vi "pionowy.vi"(6 "error in":errorcluster, 7 "Wybór komory":T1, 8 "Akcja":T8=enum."Reset ramienia", 9 "LINX Resource in":T2) -> (0 "error out":errorcluster, 1 "KONIEC":bool, 2 "Aktualny stan":T9, 3 "LINX Resource out":T2)   [LabVIEW 2014]
uses:
  pionowyVIs/RuchPionowy.ctl
  AkcjaRuchu.ctl
  <vilib>/MakerHub/LINX/Private/Type Defs/LINX Ref.ctl
  <vilib>/MakerHub/LINX/Private/Type Defs/Platform.ctl
  <vilib>/MakerHub/LINX/Private/Type Defs/Interface.ctl
  <vilib>/MakerHub/LINX/Private/Device/Type Defs/LINX Device Config.ctl
  <vilib>/MakerHub/LINX/Private/Device/Type Defs/TCP Config.ctl
  <vilib>/MakerHub/LINX/Private/Device/Type Defs/Channels.ctl
  parametryKomorVIs/WyborKomory.ctl
  Faza_ruchu.ctl
  pionowyVIs/ParametryRuchyPionowego.ctl
  pionowyVIs/usrednianieVIs/AkcjaUsredniania.ctl
  AkcjaGFV.ctl
  poziomyVIs/timerRuchuPoziomegoVIs/Czynnosc.ctl
  <vilib>/MakerHub/LINX/LMH-LINX.lvlib
  <vilib>/MakerHub/LINX/Private/Device/Device.lvlib
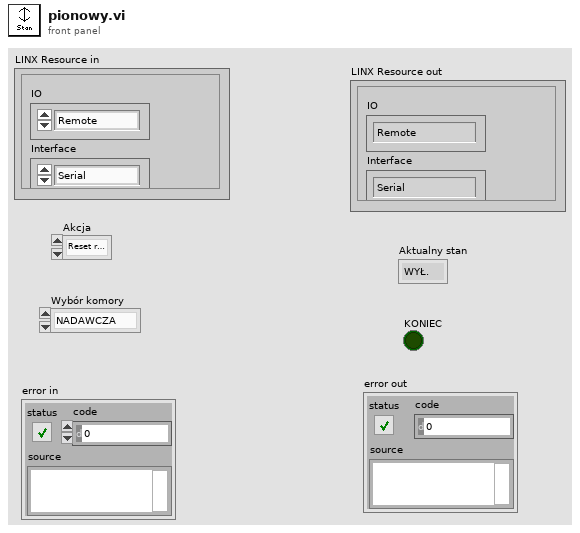
[diagram p1: front panel]
types:
  T1 = typedef "WyborKomory.ctl" = enum16{"NADAWCZA", "ODBIORCZA"}
  T2 = typedef "LMH-LINX.lvlib/LINX Ref.ctl" = cluster{"IO":T3, "Interface":T4, "LINX Device Config":T5}
  T3 = typedef "LMH-LINX.lvlib/Platform.ctl" = enum16{"Remote", "Local"}
  T4 = typedef "LMH-LINX.lvlib/Interface.ctl" = enum16{"Serial", "TCP"}
  T5 = typedef "LMH-LINX.lvlib/Device.lvlib/LINX Device Config.ctl" = cluster{"Interface":T4, "COM Port":refnum<visa-resource-name>, "TCP Configuration":T6, "Device Family":u8, "Device ID":u8, "Device Name":string, "TCP Ref":refnum<k5>, "Channels":T7}
  T6 = typedef "LMH-LINX.lvlib/Device.lvlib/TCP Config.ctl" = cluster{"IP Address":string, "Port":u16}
  T7 = typedef "LMH-LINX.lvlib/Channels.ctl" = cluster{"DI":u8[], "DO":u8[], "AI":u8[], "AO":u8[], "PWM":u8[], "QE":u8[], "UART":u8[], "I2C 2":u8[], "SPI":u8[], "CAN":u8[], "Servo":u8[], "AI Ref (V)":dbl, "AI Resolution (Bits)":u8, "AO Ref (V)":dbl, "AO Resolution (Bits)":u8}
  T8 = typedef "AkcjaRuchu.ctl" = enum16{"Init", "Reset ramienia", "Przygotuj listę", "Sprawdź", "Koniec"}
  T9 = typedef "RuchPionowy.ctl" = enum16{"WYŁ.", "GÓRA", "Dӣ", "PRACA RĘCZNA"}
  T10 = typedef "Czynnosc.ctl" = enum16{"reset all", "działaj"}
  T11 = typedef "AkcjaGFV.ctl" = enum16{"Czytaj", "Zapisz", "Reset"}
  T12 = typedef "AkcjaUsredniania.ctl" = enum16{"Init", "DodajWartość", "OdczytajPrzyspieszenie", "WypełnijKolejkę", "Czyść"}
  T13 = typedef "ParametryRuchyPionowego.ctl" = cluster{"Faza ruchu":T14, "Lista punktów w pionie":i32[]}
  T14 = typedef "Faza_ruchu.ctl" = enum16{"Ruch", "Poczekaj", "Pomiar"}
  T15 = typedef "Gotowosc.ctl" = cluster{"Poziomy":bool, "Pionowy":bool}
  T16 = typedef "WejsciaParametry.ctl" = cluster{"LEWO":bool, "PRAWO":bool, "GORA":bool, "DOL":bool, "Praca reczna":bool, "Stop":bool, "Start":bool, "Komora":bool, "Wyjscie":bool, "Rodzaj pomiarow":T17, "Czas pomiaru [s]":dbl, "Czas inicjalizacji ramion [s]":dbl, "Liczba punktów":i32, "Liczba płaszczyzn":i32}
  T17 = typedef "RodzajPomiarow.ctl" = enum16{"Izolacyjność Akustyczna ISO 10140", "Losowanie punktów", "Sekwencja testowa"}
  T18 = typedef "WyjsciaParametry.ctl" = cluster{"Nad. lewo":bool, "Nad.  prawo":bool, "Nad.  gora":bool, "Nad. doł":bool, "Dzialanie":bool, "Pomiar":bool, "Odb. lewo":bool, "Odb.  prawo":bool, "Odb.  gora":bool, "Odb. dol":bool, "Pozostalo punktow":i32, "Nad. elewacja":i32, "Nad. azymut":i32, "Odb. elewacja":i32, "Odb. azymut":i32, "TCP Error":bool, "TCP Error Code":i32, "LINX Error":bool, "LINX Error Code":i32, "Nastepny elewacja":i32, "Nastepny azymut":i32, "Coords Error":bool, "Inicjalizacja pozycji":bool}
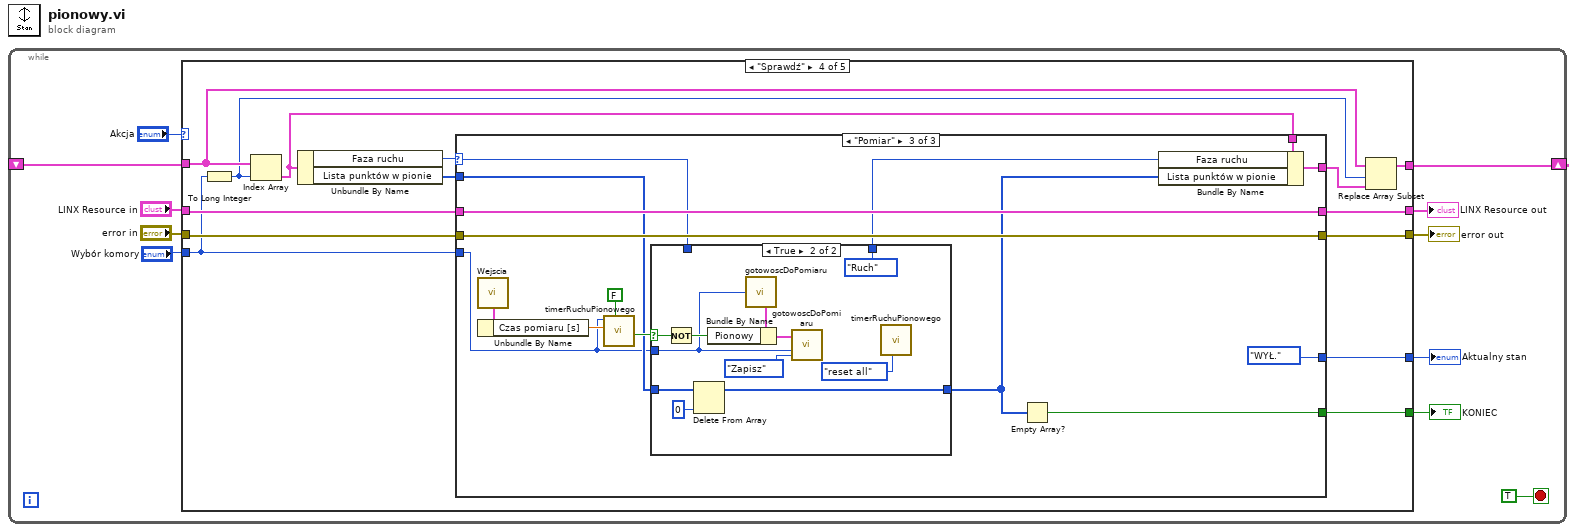
[diagram p0: block diagram]
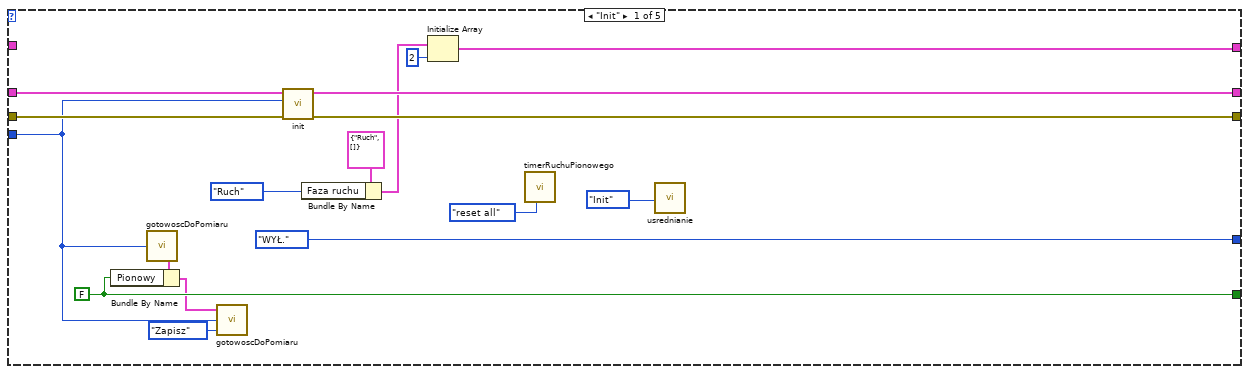
[diagram p2: hidden frame]
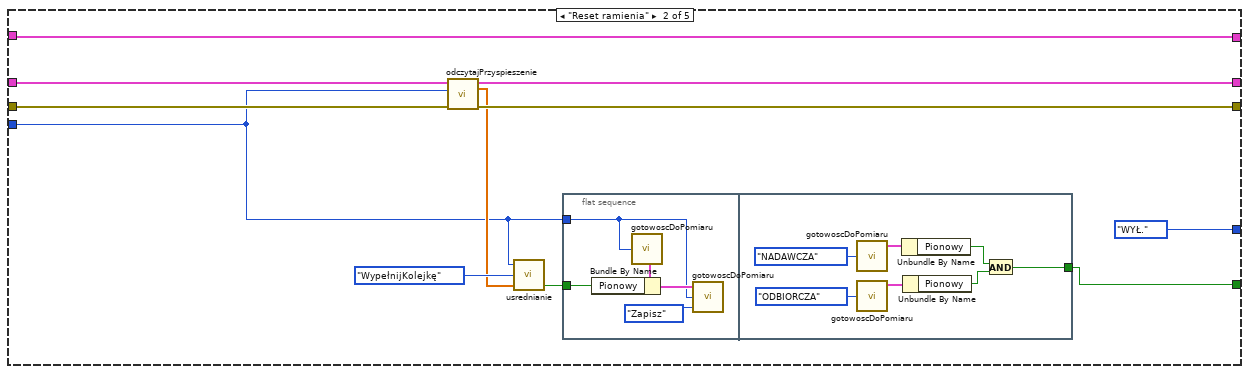
[diagram p3: hidden frame]
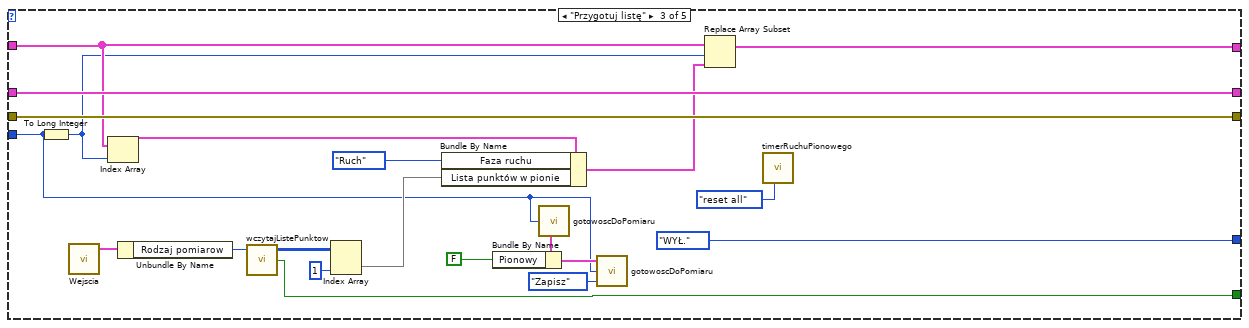
[diagram p4: hidden frame]
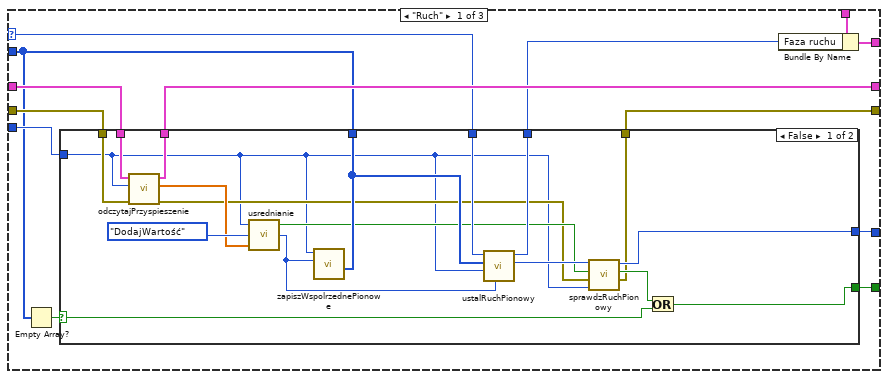
[diagram p5: hidden frame]
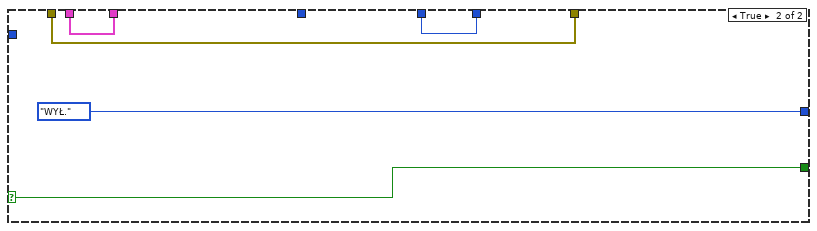
[diagram p6: hidden frame]
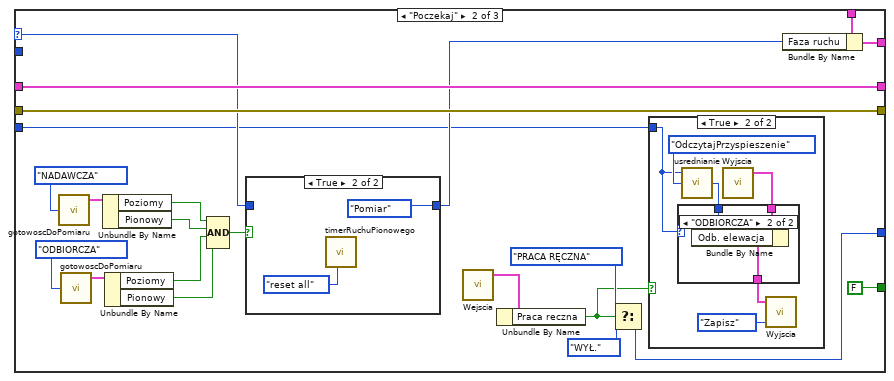
[diagram p7: hidden frame]
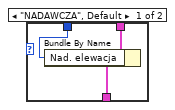
[diagram p9: hidden frame]
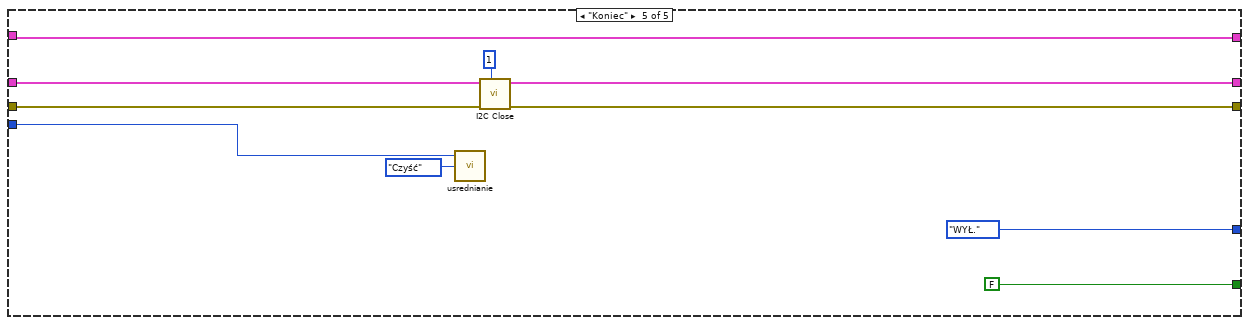
[diagram p12: hidden frame]
diagram:
  n1 = while {
    shift-right: [w10] -> _
    shift-left: _ -> [w7]
    stop <- TRUE stop-if-true
    n2 = case shown="\"Sprawdź\"" "Akcja" {
      tunnel: "error in" -> [w26 w36 w71 w85 w196]
      tunnel: [w24 w34 w71 w83 w193] -> w3
      tunnel: [w25 w35 w72 w84 w194] -> w4
      tunnel: "LINX Resource in" -> [w27 w37 w72 w86 w197]
      tunnel: [w16 w30 w53 w81 FALSE ("empty?")] -> w1
      tunnel: [RuchPionowy."WYŁ." ("Aktualny stan") RuchPionowy."WYŁ." ("Aktualny stan") RuchPionowy."WYŁ." ("Aktualny stan") w82 RuchPionowy."WYŁ." ("Aktualny stan")] -> w2
      tunnel: "Wybór komory" -> [w13 w29 w55 w80 w189]
      tunnel: [w18 w32 w68 w76 w188] -> w10
      tunnel: w7 -> [_ w32 w65 w77 w188]
      frame "Init" {
        w16 = FALSE ("Poziomy")
        n3 = call "gotowoscDoPomiaru.vi"("Wybór komory"=w13) -> ("Gotowość wyjście"=w17:T15)  [unwired: 4 in]
        n4 = Bundle By Name(cluster=w17, "Pionowy"=w16) -> (w15:T15)
        n5 = call "gotowoscDoPomiaru.vi"("Akcja"=AkcjaGFV."Zapisz", "Wybór komory"=w13, "Gotowość"=w15) -> ()  [unwired: 2 in, 1 out]
        n6 = call "init.vi"("Error In"=w26, "Wybór komory"=w13, "LINX Ref"=w27) -> ("Error Out"=w24:errorcluster, "LINX Resource"=w25:T2)  [unwired: 7 in]
        n7 = Bundle By Name(cluster=T13 {"Faza ruchu"=enum."Ruch", "Lista punktów w pionie"=[]} ("Parametry ruchy pionowego"), "Faza ruchu"=Faza_ruchu."Ruch") -> (w20:T13)
        n8 = Initialize Array(w20, 2 ("dimension size")) -> (w18:T13[])
        n9 = call "timerRuchuPionowego.vi"("Czynność"=Czynnosc."reset all") -> ()  [unwired: 10 in, 1 out]
        n10 = call "usrednianie.vi"("AkcjaUsredniania"=AkcjaUsredniania."Init") -> ()  [unwired: 2 in, 3 out]
      }
      frame "Reset ramienia" {
        n11 = call "odczytajPrzyspieszenie.vi"("Error In"=w36, "Wybór komory"=w29, "LINX Resource"=w37) -> ("Error Out"=w34:errorcluster, "Kąty nachylenia (st.)"=w33:dbl[], "LINX Resource 2"=w35:T2)  [unwired: 6 in]
        n12 = call "usrednianie.vi"("Wartości"=w33, "AkcjaUsredniania"=AkcjaUsredniania."WypełnijKolejkę", "Wybór Komory"=w29) -> ("Czy kolejka pełna?"=w31:bool)  [unwired: 2 out]
        n13 = flat-sequence {
          tunnel: w31 -> [w41]
          tunnel: w29 -> [w40]
          tunnel: [w45] -> w30
          frame #0 {
            n14 = call "gotowoscDoPomiaru.vi"("Wybór komory"=w40) -> ("Gotowość wyjście"=w44:T15)  [unwired: 4 in]
            n15 = Bundle By Name(cluster=w44, "Pionowy"=w41) -> (w43:T15)
            n16 = call "gotowoscDoPomiaru.vi"("Akcja"=AkcjaGFV."Zapisz", "Wybór komory"=w40, "Gotowość"=w43) -> ()  [unwired: 2 in, 1 out]
          }
          frame #1 {
            n17 = call "gotowoscDoPomiaru.vi"("Wybór komory"=WyborKomory."NADAWCZA") -> ("Gotowość wyjście"=w48:T15)  [unwired: 4 in]
            n18 = call "gotowoscDoPomiaru.vi"("Wybór komory"=WyborKomory."ODBIORCZA") -> ("Gotowość wyjście"=w49:T15)  [unwired: 4 in]
            n19 = Unbundle By Name(w48) -> ("Pionowy"=w51:bool)
            n20 = Unbundle By Name(w49) -> ("Pionowy"=w50:bool)
            n21 = And(x=w51, y=w50) -> (x .and. y?=w45:bool)
          }
        }
      }
      frame "Przygotuj listę" {
        n22 = To Long Integer(number=w55) -> (32bit integer=w56:i32)
        n23 = call "Wejscia.vi"() -> ("Wyjście"=w61:T16)  [unwired: 5 in]
        n24 = Index Array(array=w65, index=w56) -> (element=w66:T13)
        n25 = Unbundle By Name(w61) -> ("Rodzaj pomiarow"=w60:T17)
        n26 = call "wczytajListePunktow.vi"("Rodzaj pomiarow"=w60) -> ("Blad"=w53:bool, "Wspolrzedne katowe"=w64:i32[][])  [unwired: 3 in]
        n27 = Index Array(array=w64, index (col)=1 ("disabled index (col)")) -> (element=w62:i32[])  [unwired: 1 in]
        n28 = Bundle By Name(cluster=w66, "Faza ruchu"=Faza_ruchu."Ruch", "Lista punktów w pionie"=w62) -> (w67:T13)
        n29 = call "gotowoscDoPomiaru.vi"("Wybór komory"=w55) -> ("Gotowość wyjście"=w59:T15)  [unwired: 4 in]
        n30 = Bundle By Name(cluster=w59, "Pionowy"=FALSE ("Poziomy")) -> (w58:T15)
        n31 = call "gotowoscDoPomiaru.vi"("Akcja"=AkcjaGFV."Zapisz", "Wybór komory"=w55, "Gotowość"=w58) -> ()  [unwired: 2 in, 1 out]
        n32 = Replace Array Subset(array=w65, new element=w67, index=w56) -> (w68:T13[])
        n33 = call "timerRuchuPionowego.vi"("Czynność"=Czynnosc."reset all") -> ()  [unwired: 10 in, 1 out]
      }
      frame "Sprawdź" {
        n34 = To Long Integer(number=w80) -> (32bit integer=w74:i32)
        n35 = Index Array(array=w77, index=w74) -> (element=w73:T13)
        n36 = Unbundle By Name(w73) -> ("Faza ruchu"=w79:T14, "Lista punktów w pionie"=w78:i32[])
        n37 = case shown="\"Pomiar\"" w79 {
          selector: w79 -> [w94 w142 w169]
          tunnel: w86 -> [w98 w144 w174]
          tunnel: w85 -> [w99 w143 w173]
          tunnel: [w96 w143 w173] -> w83
          tunnel: [w97 w144 w174] -> w84
          tunnel: [w95 w139 RuchPionowy."WYŁ." ("Stan pionowy")] -> w82
          tunnel: [w92 FALSE ("empty?") w168] -> w81
          tunnel: w80 -> [w91 w123 w160]
          tunnel: w78 -> [w88 _ w167]
          tunnel: [w89 w135 w164] -> w75
          tunnel: w73 -> [w87 w134 w163]
          frame "Ruch" {
            n38 = Empty Array?(array=w88) -> (empty?=w93:bool)
            n39 = case shown="False" w93 {
              selector: w93 -> [w105 w118]
              tunnel: w99 -> [w114 w121]
              tunnel: w98 -> [w112 w122]
              tunnel: [w113 w122] -> w97
              tunnel: [w102 w121] -> w96
              tunnel: [w107 RuchPionowy."WYŁ." ("Stan pionowy")] -> w95
              tunnel: w94 -> [w116 w120]
              tunnel: [w115 w120] -> w90
              tunnel: [w104 w118] -> w92
              tunnel: w91 -> [w100 _]
              tunnel: w88 -> [w110 _]
              frame False {
                n40 = call "odczytajPrzyspieszenie.vi"("Error In"=w114, "Wybór komory"=w100, "LINX Resource"=w112) -> ("Error Out"=w103:errorcluster, "Kąty nachylenia (st.)"=w111:dbl[], "LINX Resource 2"=w113:T2)  [unwired: 6 in]
                n41 = call "usrednianie.vi"("Wartości"=w111, "AkcjaUsredniania"=AkcjaUsredniania."DodajWartość", "Wybór Komory"=w100) -> ("Kąt uśredniony"=w101:i32, "Czy nastapil krok?"=w108:bool)  [unwired: 1 out]
                n42 = call "zapiszWspolrzednePionowe.vi"("Lista punktów w pionie"=w110, "Kąt uśredniony"=w101, "Wybór komory"=w100) -> ()  [unwired: 9 in]
                n43 = call "ustalRuchPionowy.vi"("Kąt uśredniony"=w101, "Wybór komory"=w100, "Lista punktów w pionie"=w110, "Faza ruchu wstepna"=w116) -> ("Stan pionowy"=w109:T9, "Faza ruchu poziomego"=w115:T14)  [unwired: 6 in]
                n44 = call "sprawdzRuchPionowy.vi"("Wybór komory"=w100, "LINX Error IN"=w103, "Czy nastapil krok?"=w108, "Stan pionowy"=w109) -> ("LINX Error OUT"=w102:errorcluster, "KONIEC"=w106:bool, "Stan pionowy wybrany"=w107:T9)  [unwired: 5 in]
                n45 = Or(x=w106, y=w105) -> (x .or. y?=w104:bool)
              }
              frame True {
              }
            }
            n46 = Bundle By Name(cluster=w87, "Faza ruchu"=w90) -> (w89:T13)
          }
          frame "Poczekaj" {
            n47 = call "gotowoscDoPomiaru.vi"("Wybór komory"=WyborKomory."NADAWCZA") -> ("Gotowość wyjście"=w133:T15)  [unwired: 4 in]
            n48 = call "gotowoscDoPomiaru.vi"("Wybór komory"=WyborKomory."ODBIORCZA") -> ("Gotowość wyjście"=w132:T15)  [unwired: 4 in]
            n49 = Unbundle By Name(w133) -> ("Poziomy"=w131:bool, "Pionowy"=w130:bool)
            n50 = Unbundle By Name(w132) -> ("Poziomy"=w129:bool, "Pionowy"=w128:bool)
            n51 = Compound Arithmetic op=AND(w131, w130, w129, w128) -> (w125:bool)
            n52 = case shown="True" w125 {
              tunnel: w142 -> [w157 _]
              tunnel: [w157 Faza_ruchu."Pomiar" ("t")] -> w136
              frame False {
              }
              frame True {
                n53 = call "timerRuchuPionowego.vi"("Czynność"=Czynnosc."reset all") -> ()  [unwired: 10 in, 1 out]
              }
            }
            n54 = call "Wejscia.vi"() -> ("Wyjście"=w141:T16)  [unwired: 5 in]
            n55 = Unbundle By Name(w141) -> ("Praca reczna"=w124:bool)
            n56 = Select(t=RuchPionowy."PRACA RĘCZNA", s=w124, f=RuchPionowy."WYŁ." ("Stan pionowy")) -> (s? t:f=w139:T9)
            n57 = case shown="True" w124 {
              tunnel: w123 -> [_ w149]
              frame False {
              }
              frame True {
                n58 = call "usrednianie.vi"("AkcjaUsredniania"=AkcjaUsredniania."OdczytajPrzyspieszenie", "Wybór Komory"=w149) -> ("Kąt uśredniony"=w146:i32)  [unwired: 1 in, 2 out]
                n59 = call "Wyjscia.vi"() -> ("Wyjście"=w148:T18)  [unwired: 5 in]
                n60 = case shown="\"ODBIORCZA\"" w149 {
                  tunnel: [w153 w156] -> w145
                  tunnel: w148 -> [w151 w155]
                  tunnel: w146 -> [w152 w154]
                  frame "NADAWCZA", Default {
                    n61 = Bundle By Name(cluster=w151, "Nad. elewacja"=w152) -> (w153:T18)
                  }
                  frame "ODBIORCZA" {
                    n62 = Bundle By Name(cluster=w155, "Odb. elewacja"=w154) -> (w156:T18)
                  }
                }
                n63 = call "Wyjscia.vi"("Akcja"=AkcjaGFV."Zapisz", "Wejście"=w145) -> ()  [unwired: 3 in, 1 out]
              }
            }
            n64 = Bundle By Name(cluster=w134, "Faza ruchu"=w136) -> (w135:T13)
          }
          frame "Pomiar" {
            n65 = call "Wejscia.vi"() -> ("Wyjście"=w162:T16)  [unwired: 5 in]
            n66 = Unbundle By Name(w162) -> ("Czas pomiaru [s]"=w161:dbl)
            n67 = call "timerRuchuPionowego.vi"("Pauza"=FALSE ("pauza"), "Czas"=w161, "Wybór komory"=w160) -> ("Czy czas upłynął?"=w172:bool)  [unwired: 8 in]
            n68 = case shown="True" w172 {
              selector: w172 -> [_ w182]
              tunnel: [w175 w179] -> w165
              tunnel: w169 -> [w176 _]
              tunnel: [w176 Faza_ruchu."Ruch" ("Faza ruchu")] -> w166
              tunnel: w167 -> [w175 w183]
              tunnel: w160 -> [_ w177]
              frame False {
              }
              frame True {
                n69 = Not(x=w182) -> (.not. x?=w181:bool)
                n70 = Delete From Array(array=w183, index=0) -> (array with subset deleted=w179:i32[])  [unwired: 1 in, 1 out]
                n71 = call "gotowoscDoPomiaru.vi"("Wybór komory"=w177) -> ("Gotowość wyjście"=w184:T15)  [unwired: 4 in]
                n72 = Bundle By Name(cluster=w184, "Pionowy"=w181) -> (w185:T15)
                n73 = call "gotowoscDoPomiaru.vi"("Akcja"=AkcjaGFV."Zapisz", "Wybór komory"=w177, "Gotowość"=w185) -> ()  [unwired: 2 in, 1 out]
                n74 = call "timerRuchuPionowego.vi"("Czynność"=Czynnosc."reset all") -> ()  [unwired: 10 in, 1 out]
              }
            }
            n75 = Empty Array?(array=w165) -> (empty?=w168:bool)
            n76 = Bundle By Name(cluster=w163, "Faza ruchu"=w166, "Lista punktów w pionie"=w165) -> (w164:T13)
          }
        }
        n77 = Replace Array Subset(array=w77, new element=w75, index=w74) -> (w76:T13[])
      }
      frame "Koniec" {
        n78 = call "usrednianie.vi"("AkcjaUsredniania"=AkcjaUsredniania."Czyść", "Wybór Komory"=w189) -> ()  [unwired: 1 in, 3 out]
        n79 = call <vilib>:"I2C Close.vi"("I2C Channel (0)"=u8 1, "Error In"=w196, "LINX Resource"=w197) -> ("Error Out"=w193:errorcluster, "LINX Resource"=w194:T2)  [unwired: 7 in]
      }
    }
    "error out" <- w3
    "LINX Resource out" <- w4
    "KONIEC" <- w1
    "Aktualny stan" <- w2
  }
